vi "Stop.vi"(8 "Error In":errorcluster, 11 "object in":refnum<class "PXI-5441.lvclass">) -> (0 "Error Out":errorcluster, 3 "object out":refnum<class "PXI-5441.lvclass">)   [LabVIEW 2023, in "PXI-5441.lvlib" / "PXI-5441.lvclass"]
uses:
  PXI-5441.lvclass
  PXI-5441.lvclass/PXI-5441.ctl
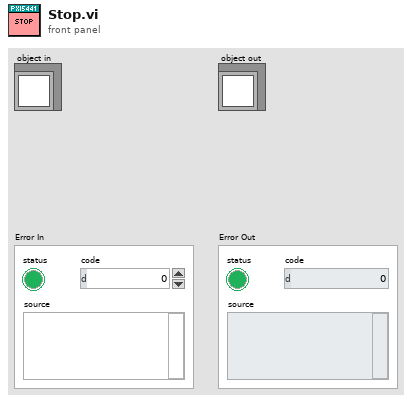
[diagram p1: front panel]
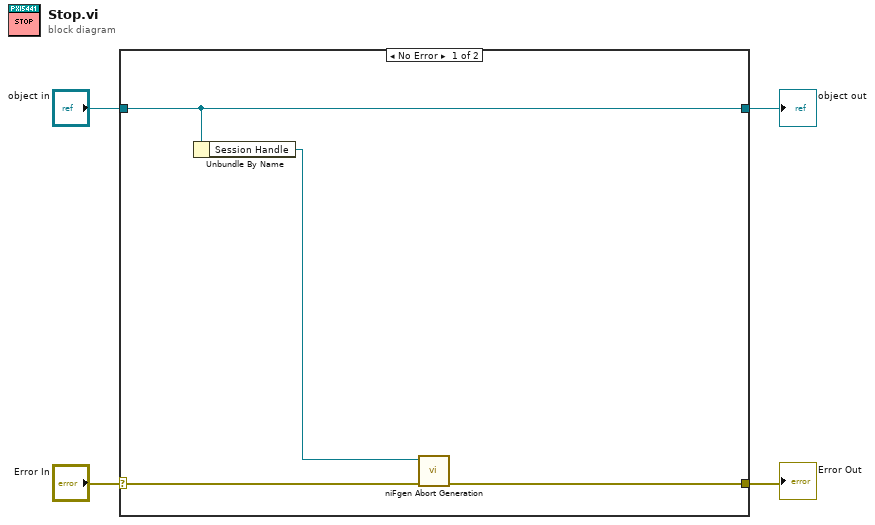
[diagram p0: block diagram]
diagram:
  n1 = case shown="No Error" "Error In" {
    selector: "Error In" -> [w8 w10]
    tunnel: [w6 w10] -> w3
    tunnel: [w7 w9] -> w1
    tunnel: "object in" -> [w7 w9]
    frame No Error {
      n2 = Unbundle By Name(w7) -> ("Session Handle"=w5:refnum<k15>)
      n3 = call <instrlib>:"niFgen Abort Generation.vi"("error in (no error)"=w8, "Instrument Handle"=w5) -> ("error out"=w6:errorcluster)  [unwired: 8 in, 1 out]
    }
    frame Error {
    }
  }
  "Error Out" <- w3
  "object out" <- w1
